vi "LoadImbalance.vi"(1 "C":dbl, 2 "B":dbl, 3 "A":dbl) -> (0 "Load Imbalance":dbl format="%0.2f")   [LabVIEW 2013]
uses:
  <vilib>/ptbypt/NI_PtbyPt.lvlib
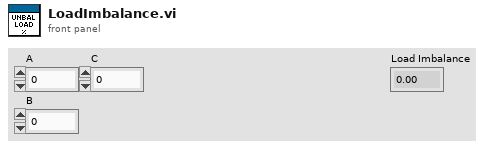
[diagram p1: front panel]
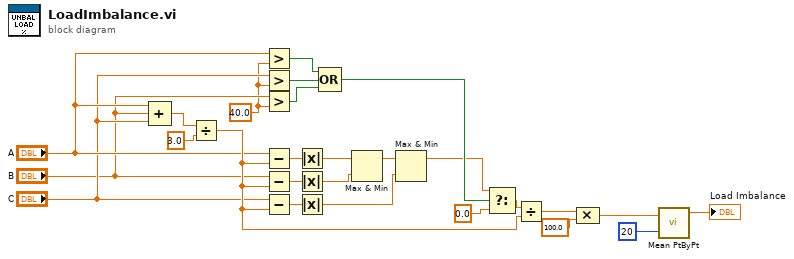
[diagram p0: block diagram]
diagram:
  w1 = 40.0
  n1 = Compound Arithmetic op=ADD("A", "B", "C") -> (w25:dbl)
  n2 = Divide(x=w25, y=3.0) -> (x/y=w12:dbl)
  n3 = Greater?(x="A", y=w1) -> (0:w8:bool)
  n4 = Greater?(x="C", y=w1) -> (0:w7:bool)
  n5 = Greater?(x="B", y=w1) -> (0:w6:bool)
  n6 = Subtract(x="A", y=w12) -> (x-y=w24:dbl)
  n7 = Subtract(x="B", y=w12) -> (x-y=w23:dbl)
  n8 = Subtract(x="C", y=w12) -> (x-y=w22:dbl)
  n9 = Absolute Value(x=w24) -> (abs(x)=w21:dbl)
  n10 = Absolute Value(x=w23) -> (abs(x)=w20:dbl)
  n11 = Absolute Value(x=w22) -> (abs(x)=w18:dbl)
  n12 = Compound Arithmetic op=OR(w8, w7, w6) -> (w4:bool)
  n13 = Max & Min(x=w21, y=w20) -> (max(x,y)=w19:dbl)  [unwired: 1 out]
  n14 = Max & Min(x=w19, y=w18) -> (max(x,y)=w3:dbl)  [unwired: 1 out]
  n15 = Select(t=w3, s=w4, f=0.0) -> (s? t:f=w5:dbl)
  n16 = Divide(x=w5, y=w12) -> (x/y=w17:dbl)
  n17 = Compound Arithmetic op=MULTIPLY(w17, 100.0 ("value")) -> (w14:dbl)
  n18 = call <vilib>:"Mean PtByPt.vi"("x"=w14, "sample length"=20) -> ("mean"=→"Load Imbalance":dbl)  [unwired: 2 in, 1 out]
